vi "JKISM++ State Table - DebugTool.vi"() -> ()   [LabVIEW 2014]
uses:
  _Support/Typedef/_JKISM Current State.ctl
  _Polymophic/Add State(s) to Queue By BOOL(Element).vi
  _Support/GlobalEvent/FGV-GlobalEventRef.vi
  <resource>/dialog/lvconfig.llb/LV Config Write Numeric (I32).vi
  <resource>/dialog/lvconfig.llb/LV Config Read Numeric (I32).vi
  _Support/jkism-tool-support.lvlib
  JKI State Machine++.lvlib
panel:
  in  "Clear JKISM":bool
  out "Dashboard":T1(array[cluster])
  out "Table Control":string[][](table)
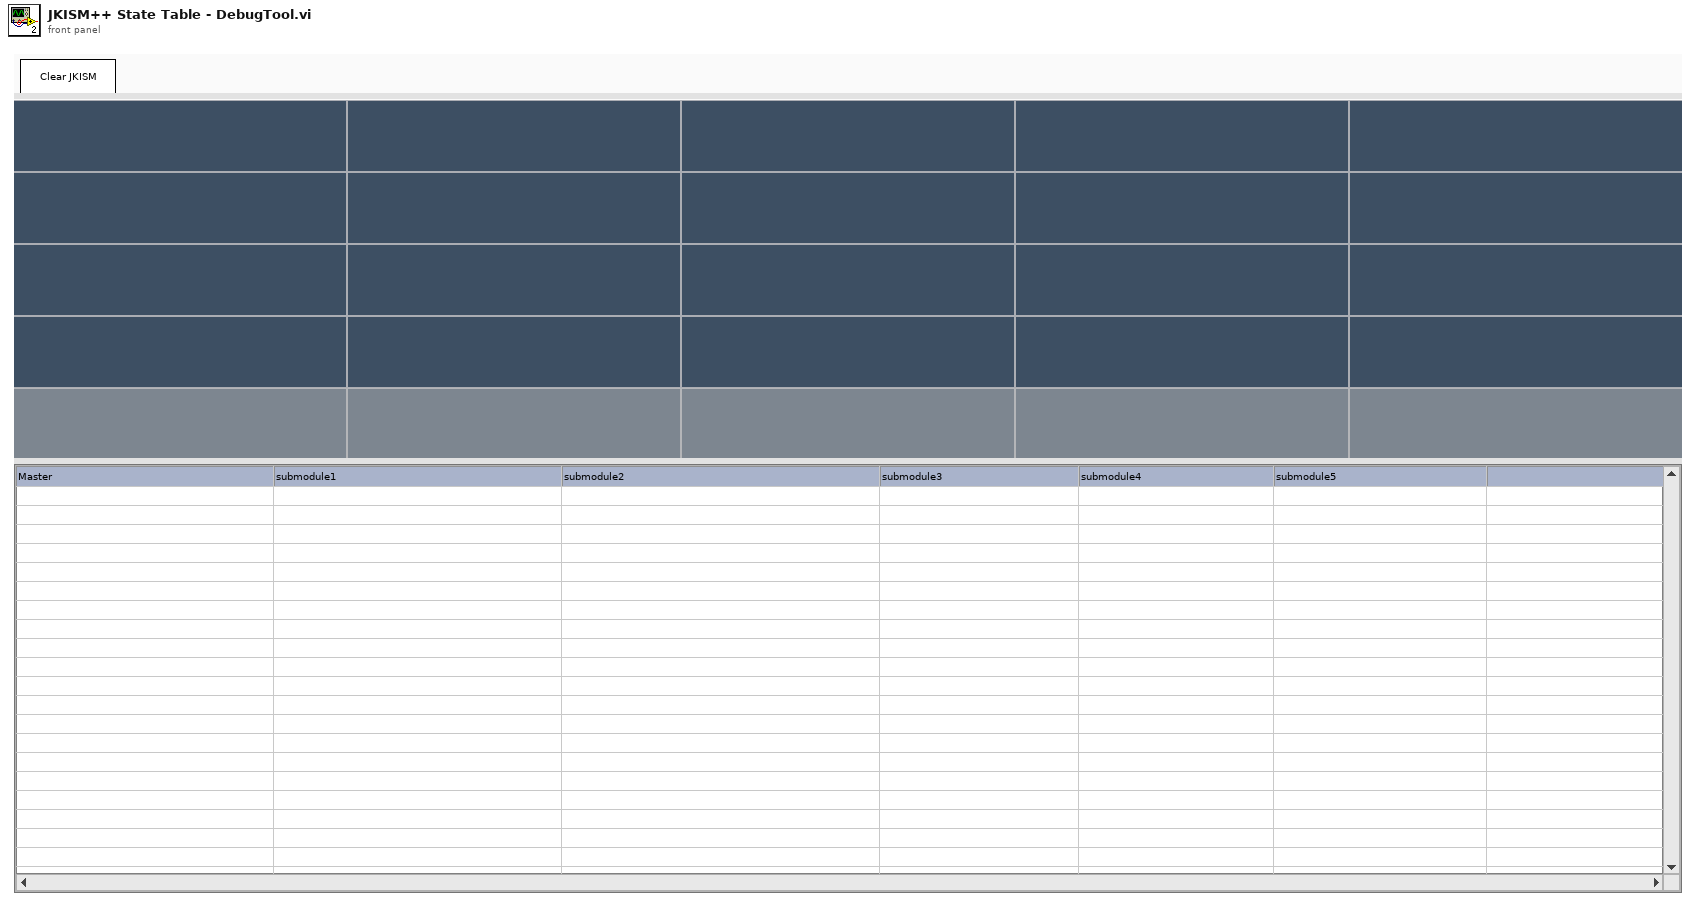
[diagram p1: front panel]
types:
  T1 = cluster{"Label":string, "Value":string, "String":string}[][]
  T2 = enum32{"Invalid", "Standard", "Closed", "Hidden", "Minimized", "Maximized"}
  T3 = enum32{"invalid app kind", "Development System", "Run Time System", "Student Edition", "Embedded LabVIEW", "Evaluation", "Custom"}
  T4 = typedef "JKI State Machine++.lvlib/_JKISM Current State.ctl" = cluster{"Name(\"\" to use uuid)":string, "Current State":string, "Arguments":string, "Argument - State":string, "From Who":string, "Complete(T)/Start(F)":bool}
  T5 = cluster{"Label":string, "Value":string, "String":string}
  T6 = cluster{"Core":cluster{"Current VI Reference":refnum<vi>, "Close Panel on Exit?":bool}, "Global-DataTable":string[][], "NumCols":i16, "NumRows":i16, "JKISM Global Log Event":refnum<user-event>, "Log":T4, "JKISM Names":string[]}
  T7 = cluster{"Current VI Reference":refnum<vi>, "Close Panel on Exit?":bool}
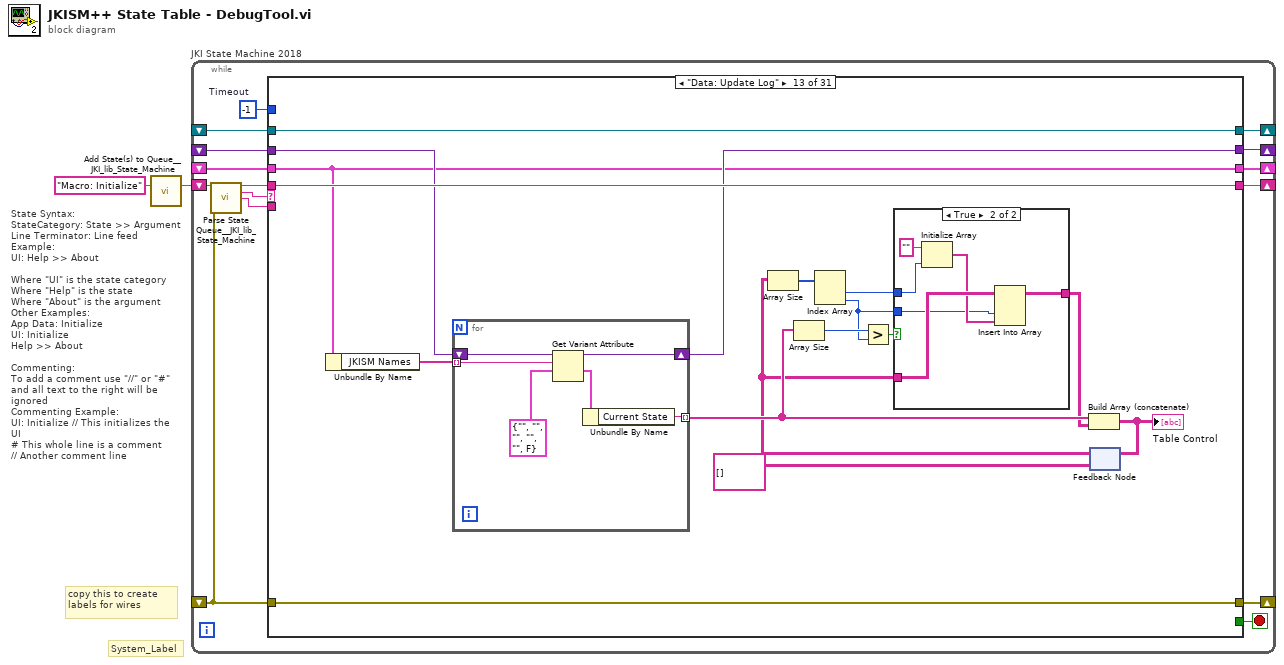
[diagram p0: block diagram]
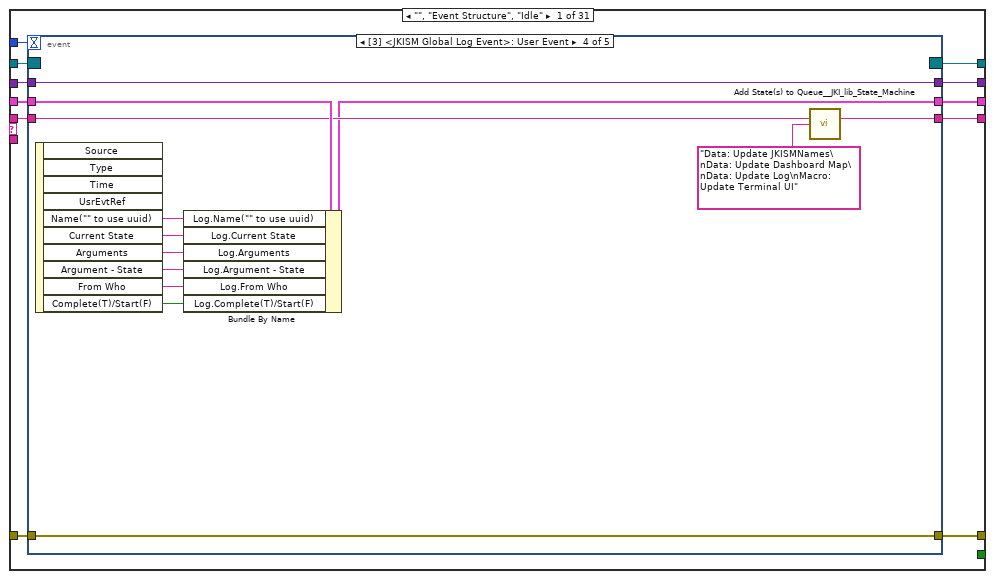
[diagram p2: hidden frame]
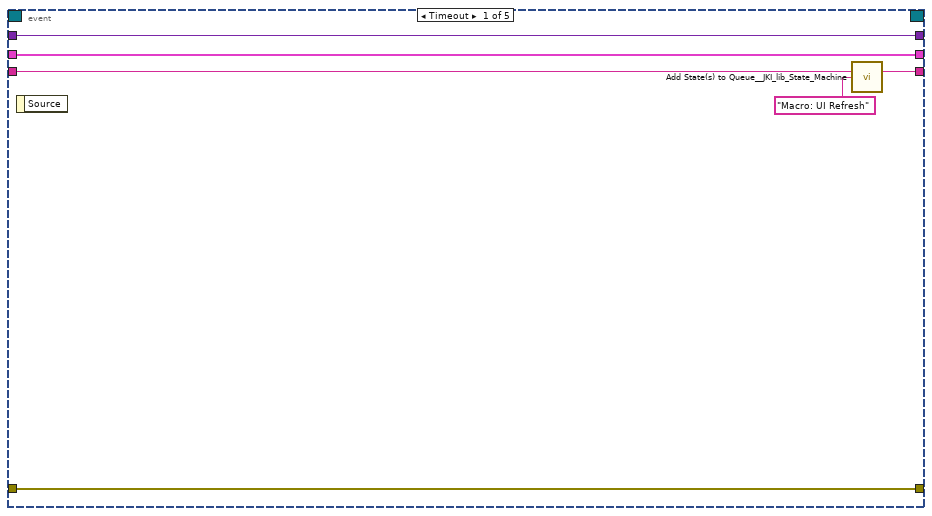
[diagram p3: hidden frame]
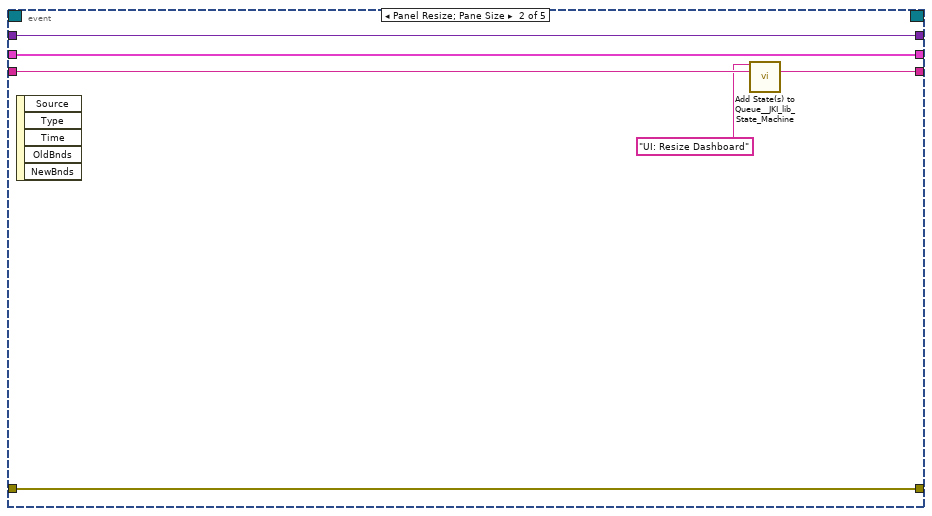
[diagram p4: hidden frame]
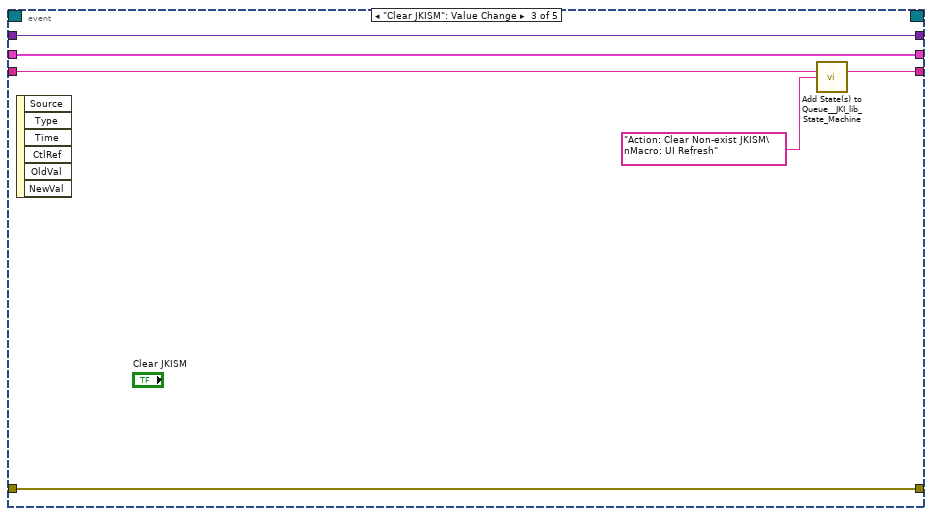
[diagram p5: hidden frame]
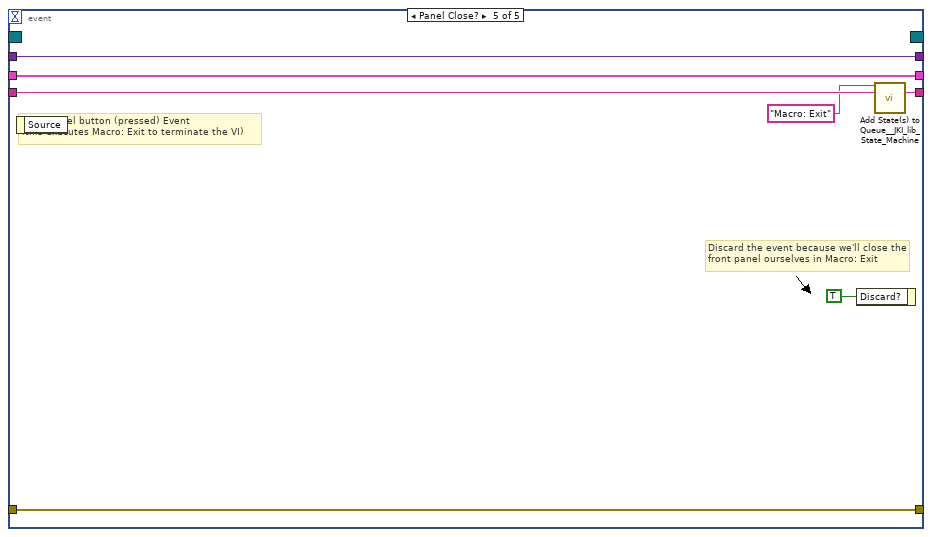
[diagram p6: hidden frame]
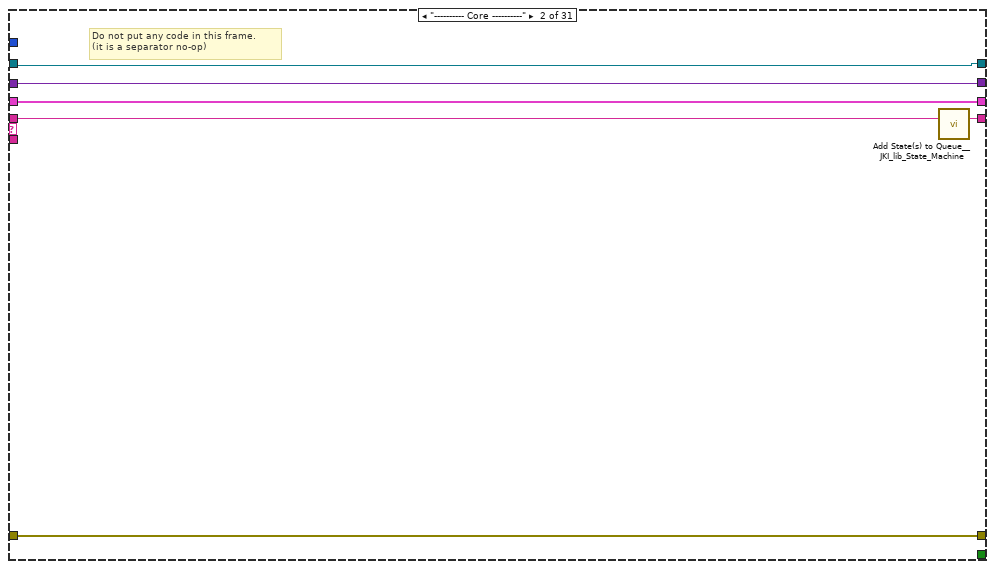
[diagram p7: hidden frame]
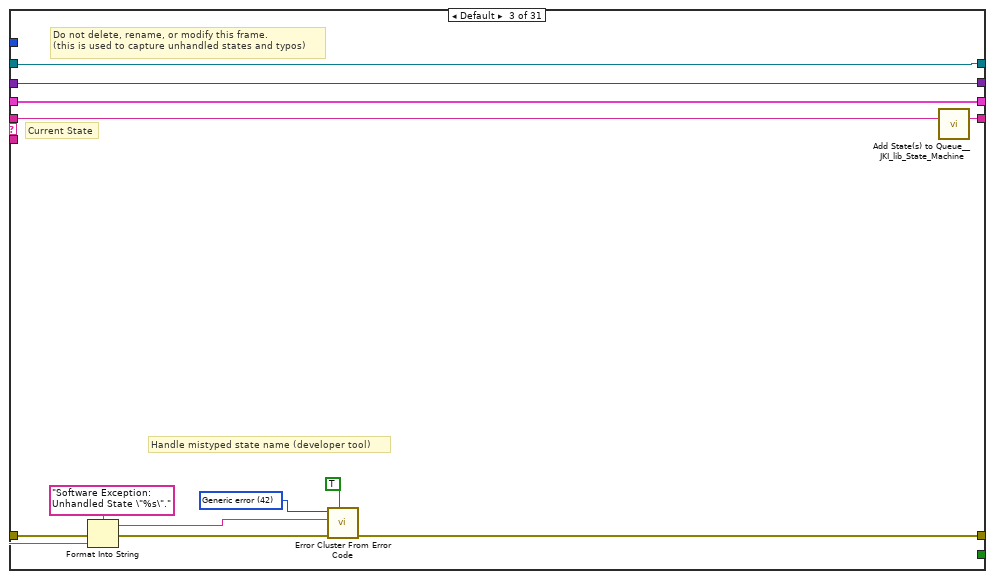
[diagram p8: hidden frame]
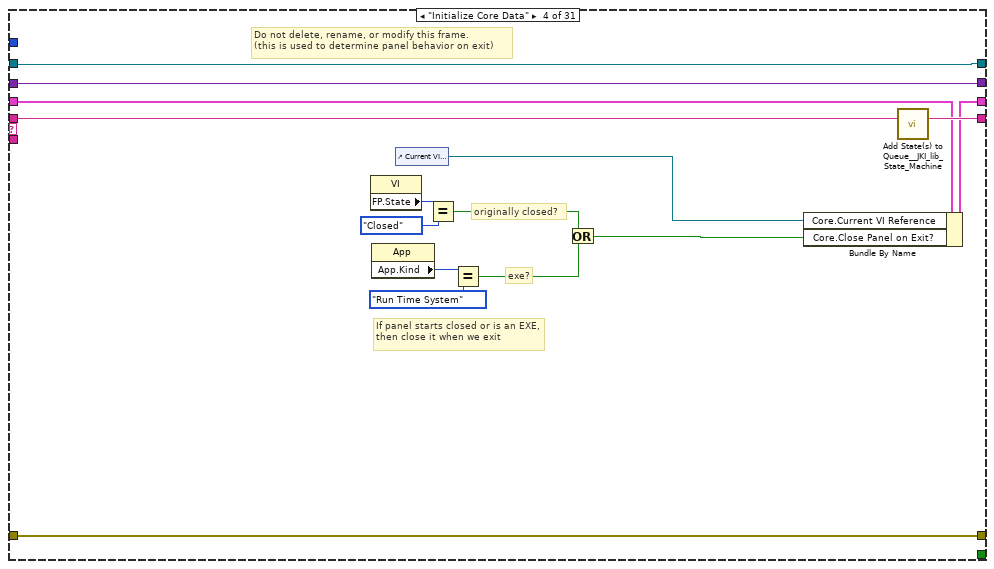
[diagram p9: hidden frame]
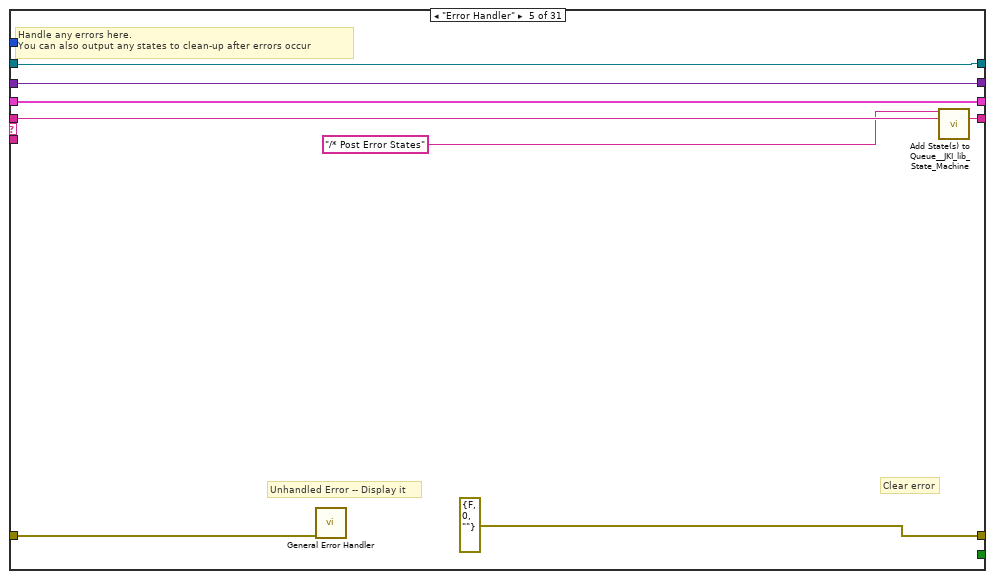
[diagram p10: hidden frame]
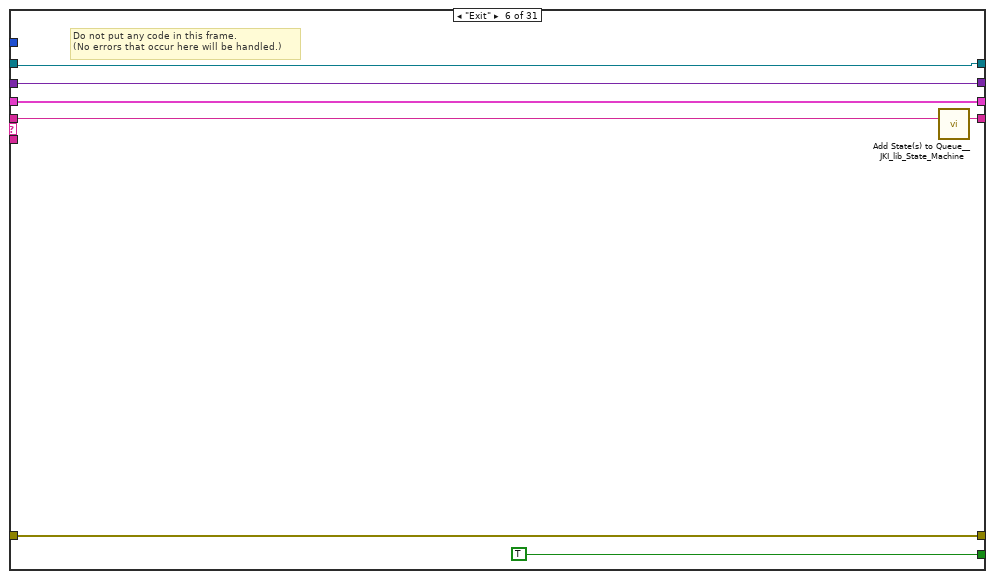
[diagram p11: hidden frame]
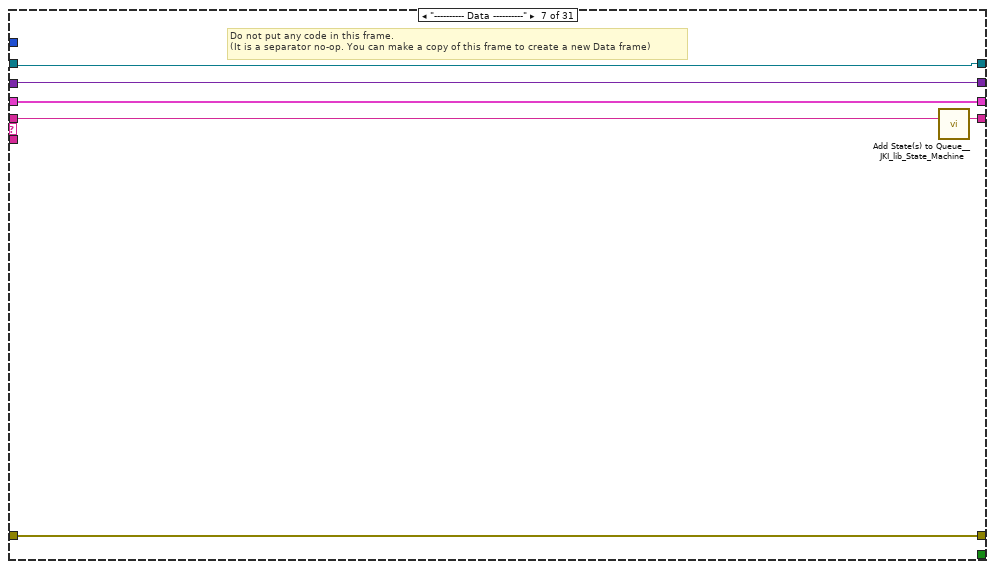
[diagram p12: hidden frame]
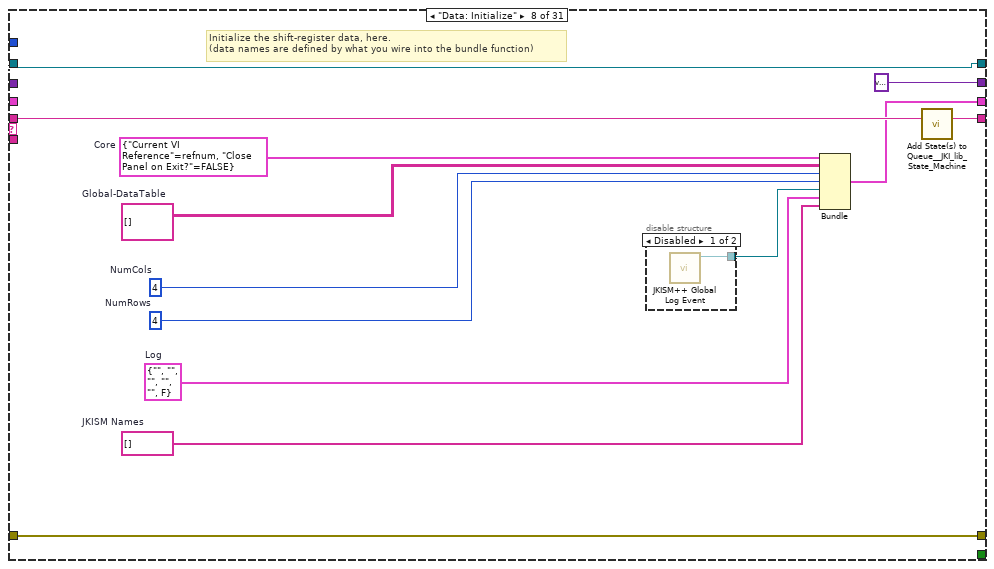
[diagram p13: hidden frame]
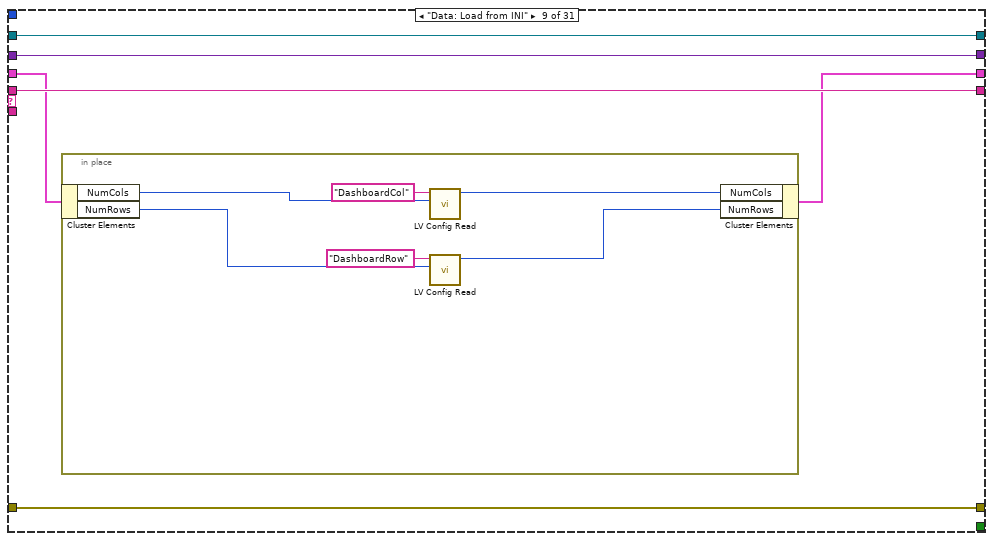
[diagram p15: hidden frame]
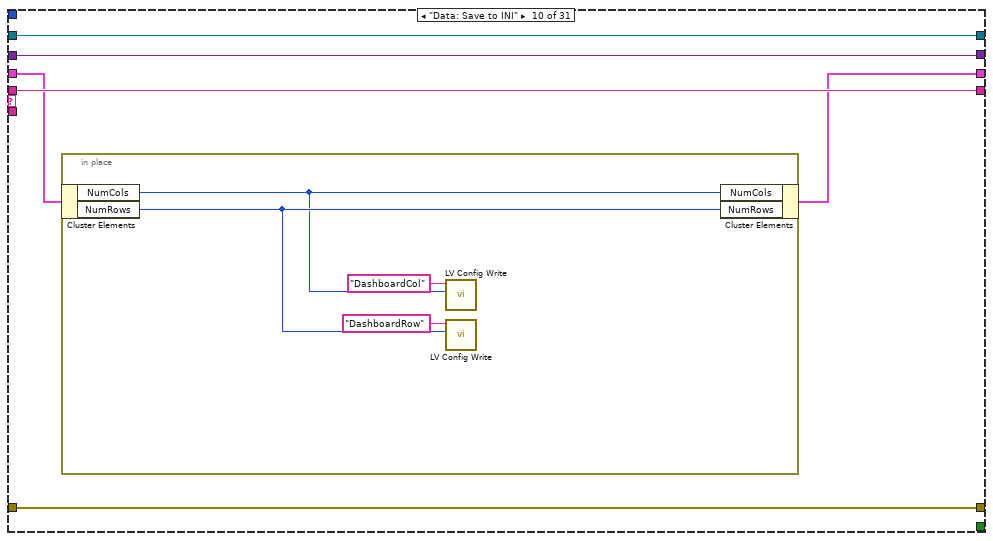
[diagram p16: hidden frame]
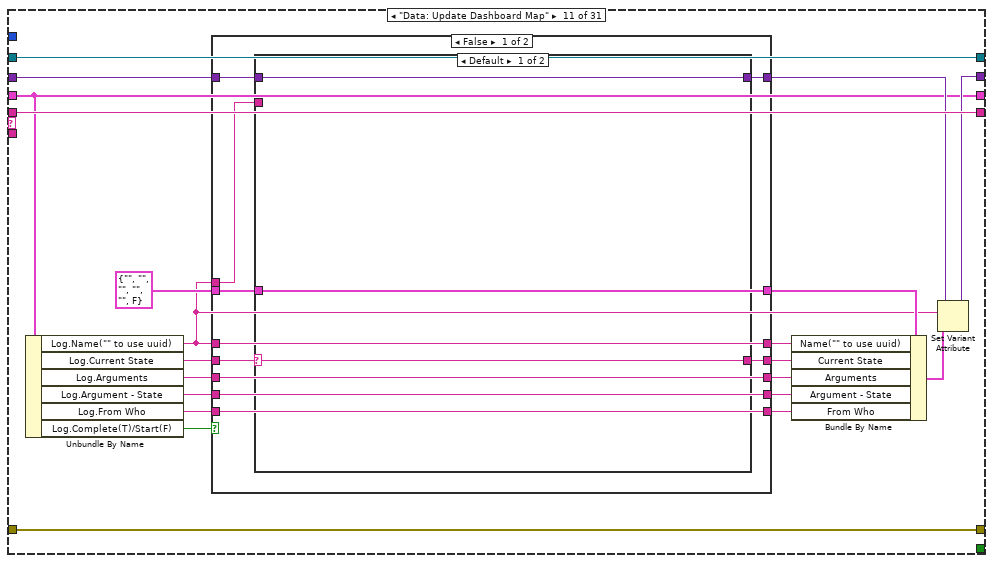
[diagram p17: hidden frame]
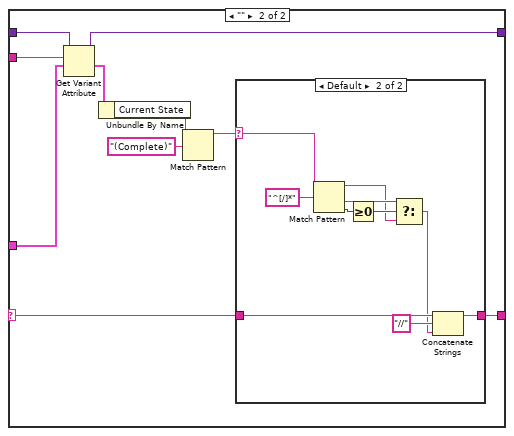
[diagram p18: hidden frame]
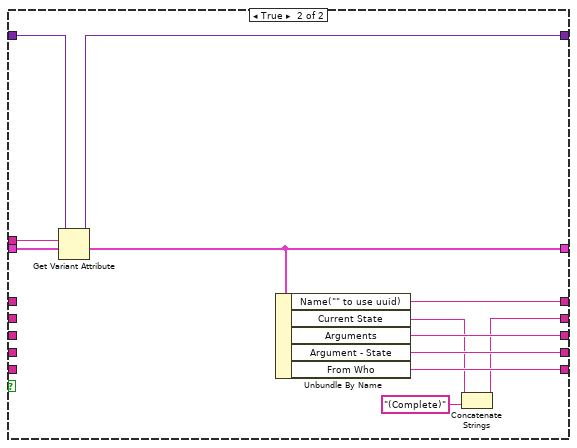
[diagram p20: hidden frame]
diagram:
  # "State Syntax:\nStateCategory: State >> Argument\nLine Terminator: Line feed\nExample:\nUI: Help >> About\n\nWhere \"UI\" is the state category\nWhere \"Help\" is the state\nWhere \"About\" is the argument\nOther Examples:\nApp Data: Initialize\nUI: Initialize\nHelp >> About\n\nCommenting:\nTo add a comment use \"//\" or \"#\" and all text to the right will be ignored\nCommenting Example:\nUI: Initialize // This initializes the UI\n# This whole line is a comment\n// Another comment line"
  # "copy this to create labels for wires"
  # "System_Label"
  n1 = call <vilib>:"Add State(s) to Queue__JKI_lib_State_Machine.vi"("State(s) in (\"\")"="Macro: Initialize") -> ("States Out"=w1:string)  [unwired: 14 in]
  n2 = while "JKI State Machine 2018" {
    shift-right: [w10] -> _
    shift-left: _ -> [w9]
    shift-right: [w13] -> _
    shift-left: _ -> [w7]
    shift-right: [w12] -> _
    shift-left: w1 -> [w14]
    shift-right: [w6] -> _
    shift-left: _ -> [w5]
    shift-right: [w4] -> _
    shift-left: _ -> [w3]
    stop <- w11 stop-if-true
    w8 = -1  # Timeout
    n3 = call <vilib>:"Parse State Queue__JKI_lib_State_Machine.vi"("State Queue"=w14, "Error In (no error)"=w7) -> ("Remaining States"=w16:string, "Current State"=w17:string, "Arguments"=w15:string)  [unwired: 11 in]
    n4 = case shown="\"Data: Update Log\"" w17 {
      selector: w17 -> [_ _ w75 _ _ _ _ _ _ _ _ _ _ _ _ _ _ _ _ _ _ _ _ _ _ _ _ _ _ _ _]
      tunnel: w16 -> [w28 w72 w79 w100 w108 w115 w121 w134 w140 w152 w177 w234 w257 w280 w286 w295 w307 w320 w397 w412 w423 w428 w436 w444 w451 w458 w466 w473 w486 w490 w501]
      tunnel: w15 -> [_ _ _ _ _ _ _ _ _ _ _ _ _ _ _ _ w302 w314 _ _ _ _ _ _ _ _ _ _ _ _ _]
      tunnel: w9 -> [w26 w69 w77 w93 w105 w113 w118 _ w139 w151 w164 w228 w253 w275 w283 w291 w305 w316 w393 w409 w420 w427 w435 w440 w448 w455 w461 w470 w483 w489 w500]
      tunnel: [w25 w70 w81 w97 errorcluster {"status"=FALSE, "code"=0, "source"=""} ("error out") w112 w119 w130 w141 w153 w178 w235 w258 w274 w284 w293 w303 w317 w394 w410 w424 w429 w437 w445 w449 w456 w464 w471 w484 w491 w502] -> w13
      tunnel: w7 -> [w24 w70 w80 w97 w104 w112 w119 w130 w141 w153 w178 w235 w258 w277 w284 w293 w304 w318 _ w410 w424 w429 w437 w445 w449 w456 w464 w471 w484 w491 w502]
      tunnel: [w27 w71 w78 w99 w107 w114 w120 w133 w140 w152 w177 w226 w257 w279 w285 w294 w306 w319 w396 w411 w423 w428 w436 w444 w450 w457 w465 w472 w485 w490 w501] -> w12
      tunnel: [_ _ _ _ _ TRUE _ _ _ _ _ _ _ _ _ _ _ _ _ _ _ _ _ _ _ _ _ _ _ _ _] -> w11
      tunnel: [w23 w69 w77 w98 w105 w113 w118 w132 w138 w150 w164 w227 w253 w275 w283 w291 w305 w316 w393 w409 w420 w427 w431 w440 w448 w455 w461 w470 w483 w489 w500] -> w10
      tunnel: w8 -> [w22 _ _ _ _ _ _ _ _ _ _ _ _ _ _ _ _ _ _ _ _ _ _ _ _ _ _ _ _ _ _]
      tunnel: [w20 w68 w74 w87 w102 w110 w117 variant w137 w149 w165 w232 w254 w273 w282 w288 w301 w313 w390 w404 w422 w426 w434 w443 w447 w453 w460 w468 w476 w488 w496] -> w6
      tunnel: w5 -> [w21 w68 w74 w87 w102 w110 w117 _ w137 w149 w166 w230 w255 w273 w282 w288 w301 w313 w390 w403 w422 w426 w434 w443 w447 w453 w460 w468 w476 w488 w498]
      tunnel: [w18 w67 w73 w86 w101 w109 w116 w125 w136 w148 w176 w233 w256 w272 w281 w287 w300 w312 w389 w400 w421 w425 w432 w442 w446 w452 w459 w467 w475 w487 w499] -> w4
      tunnel: w3 -> [w19 w67 w73 w86 w101 w109 w116 w125 w136 w148 w176 w233 w256 w272 w281 w287 w300 w312 w389 w400 w421 w425 _ w442 w446 w452 w459 w467 w475 w487 w499]
      frame "", "Event Structure", "Idle" {
        n5 = event shown="[3] <JKISM Global Log Event>: User Event" {
          selector: w19 -> [_ _ _ _ _]
          dyn-events: [_ _ _ _ _] -> w18
          timeout: w22 -> [_ _ _ _ _]
          tunnel: w28 -> [w34 w37 w43 w54 w66]
          tunnel: [w33 w38 w42 w58 w65] -> w27
          tunnel: w26 -> [w31 w39 w45 w55 w64]
          tunnel: [w32 w40 w46 w59 w61] -> w25
          tunnel: w24 -> [w32 w40 w46 w59 w61]
          tunnel: [w31 w39 w45 w53 w64] -> w23
          tunnel: w21 -> [w29 w35 w44 w56 w60]
          tunnel: [w29 w35 w44 w56 w60] -> w20
          event Timeout {
            n6 = event-data() -> ()  [unwired: 1 in, 1 out]
            n7 = call <vilib>:"Add State(s) to Queue__JKI_lib_State_Machine.vi"("State(s) in (\"\")"=w34, "State(s) at Back (\"\")"="Macro: UI Refresh" ("State(s) in Front (\"\")")) -> ("States Out"=w33:string)  [unwired: 13 in]
          }
          event Panel Resize; Pane Size {
            n8 = event-data() -> ()  [unwired: 1 in, 5 out]
            n9 = call <vilib>:"Add State(s) to Queue__JKI_lib_State_Machine.vi"("State(s) in Front (\"\")"="UI: Resize Dashboard" ("State(s) in Front (\"\")"), "State(s) in (\"\")"=w37) -> ("States Out"=w38:string)  [unwired: 13 in]
          }
          event "Clear JKISM": Value Change {
            n10 = event-data() -> ()  [unwired: 1 in, 6 out]
            n11 = call <vilib>:"Add State(s) to Queue__JKI_lib_State_Machine.vi"("State(s) in (\"\")"=w43, "State(s) at Back (\"\")"="Action: Clear Non-exist JKISM\nMacro: UI Refresh" ("State(s) at Back (\"\")")) -> ("States Out"=w42:string)  [unwired: 13 in]
          }
          event User Event {
            n12 = event-data() -> ("Name(\"\" to use uuid)"=w47:string, "Current State"=w48:string, "Arguments"=w49:string, "Argument - State"=w50:string, "From Who"=w51:string, "Complete(T)/Start(F)"=w52:bool)  [unwired: 1 in, 4 out]
            n13 = Bundle By Name(cluster=w55, "Log.Name(\"\" to use uuid)"=w47, "Log.Current State"=w48, "Log.Arguments"=w49, "Log.Argument - State"=w50, "Log.From Who"=w51, "Log.Complete(T)/Start(F)"=w52) -> (w53:T6)
            n14 = call <vilib>:"Add State(s) to Queue__JKI_lib_State_Machine.vi"("State(s) in (\"\")"=w54, "State(s) at Back (\"\")"="Data: Update JKISMNames\nData: Update Dashboard Map\nData: Update Log\nMacro: Update Terminal UI" ("State(s) at Back (\"\")")) -> ("States Out"=w58:string)  [unwired: 13 in]
          }
          event Panel Close? {
            # "Discard the event because we'll close the front panel ourselves in Macro: Exit"
            # "Close Panel button (pressed) Event\n(this executes Macro: Exit to terminate the VI)"
            n15 = event-data() -> ()  [unwired: 1 in, 1 out]
            n16 = event-data("Discard?"=TRUE) -> ()  [unwired: 1 in, 1 out]
            n17 = call <vilib>:"Add State(s) to Queue__JKI_lib_State_Machine.vi"("State(s) in Front (\"\")"="Macro: Exit", "State(s) in (\"\")"=w66) -> ("States Out"=w65:string)  [unwired: 13 in]
          }
        }
      }
      frame "---------- Core ----------" {
        # "Do not put any code in this frame.\n(it is a separator no-op)"
        n18 = call <vilib>:"Add State(s) to Queue__JKI_lib_State_Machine.vi"("State(s) in (\"\")"=w72) -> ("States Out"=w71:string)  [unwired: 14 in]
      }
      frame Default {
        w84 = 42 items=["No error", "Argument error", "Memory is full", "Out of zone", "End of file", "File already open", "Generic file I/O error", "File not found", "File permission error", "Disk is full", "Duplicate path", "Too many files open", "System feature not enabled", "Resource file not found", "Cannot add resource", "Resource not found", "Image not found", "Image memory error", "Pen does not exist", "Config type invalid", "Config token not found", "Config parse error", "Config memory error", "Bad external code format", "Bad external code offset", "External code not present", "Null window", "Destroy window error", "Null menu", "Print aborted", "Bad print record", "Print driver error", "Windows error during printing", "Memory error during printing", "Print dialog error", "Generic print error", "Invalid device refnum", "Device not found", "Device parameter error", "Device unit error", "Cannot open device", "Device call aborted", "Generic error", "Cancelled by user", "Object ID too low", "Object ID too high", "Object not in heap", "Unknown heap", "Unknown object (invalid DefProc)", "Unknown object (DefProc not in table)", "Message out of range", "Invalid (null) method", "Unknown message", "Manager call not supported", "Bad address", "Network operation in progress", "Network operation timed out", "Connection is busy", "Network attribute not supported", "Network error", "Address in use", "System out of memory", "Connection aborted", "Connection refused", "Not connected", "Already connected", "Connection closed", "Initialization error (interapplication manager)", "Bad occurrence", "Wait on unbound occurrence handler", "Occurrence queue overflow", "Datalog type conflict", "Unused", "Unrecognized type (interapplication manager)", "Memory corrupt", "Failed to make temporary DLL", "Old CIN version", "Drag socket not found", "Failed to load drop-object", "Failed to register OLE object", "Failed to release OLE object", "Format specifier type mismatch", "Unknown format specifier", "Too few format specifiers", "Too many format specifiers", "Scan failed", "Newer CIN version", "Error converting to variant", "Runtime menu error", "Password tampered", "Variant attribute not found", "Incompatible variant data type", "Event data is not available", "Event Store is not present", "Occurrence is not found", "Event Queue is not created", "Event info is not available", "Refnum passed is NULL", "Error retrieving Class GUID", "Error retrieving CoClass GUID", "Error retrieving TypeLib GUID.", "Bad built application magic bytes.", "Specific driver is different from the specific driver associated with the Logical Name.", "There is no session opened to the class driver.", "Max Error", "MAX - Error with config objects", "MAX - Error loading configuration", "MAX - Group not supported"]
        # "Current State"
        # "Do not delete, rename, or modify this frame.\n(this is used to capture unhandled states and typos)"
        # "Handle mistyped state name (developer tool)"
        n19 = Format Into String(format string="Software Exception: Unhandled State \"%s\"." ("message"), error in=w80, w75) -> (resulting string=w83:string, error out=w82:errorcluster)  [unwired: 1 in]
        n20 = call <vilib>:"Error Cluster From Error Code.vi"("show call chain? (False)"=TRUE, "error in (no error)"=w82, "error message (\"\")"=w83, "error code (0)"=w84) -> ("error out"=w81:errorcluster)  [unwired: 5 in]
        n21 = call <vilib>:"Add State(s) to Queue__JKI_lib_State_Machine.vi"("State(s) in (\"\")"=w79) -> ("States Out"=w78:string)  [unwired: 14 in]
      }
      frame "Initialize Core Data" {
        # "Do not delete, rename, or modify this frame.\n(this is used to determine panel behavior on exit)"
        # "originally closed?"
        # "exe?"
        # "If panel starts closed or is an EXE, then close it when we exit"
        n22 = property class="VI"() -> ("FP.State"=w90:T2)  [unwired: 2 in, 2 out]
        n23 = property class="App"() -> ("App.Kind"=w96:T3)  [unwired: 2 in, 2 out]
        n24 = control-ref of="Current VI Reference"() -> (w91:refnum<vi>)
        n25 = Equal?(x=w90, y=T2."Closed" ("Front Panel Window:State")) -> (x = y?=w88:bool)
        n26 = Equal?(x=w96, y=T3."Run Time System" ("Application:Kind")) -> (x = y?=w94:bool)
        n27 = Or(x=w88, y=w94) -> (x .or. y?=w92:bool)
        n28 = Bundle By Name(cluster=w93, "Core.Current VI Reference"=w91, "Core.Close Panel on Exit?"=w92) -> (w98:T6)
        n29 = call <vilib>:"Add State(s) to Queue__JKI_lib_State_Machine.vi"("State(s) in (\"\")"=w100) -> ("States Out"=w99:string)  [unwired: 14 in]
      }
      frame "Error Handler" {
        # "Unhandled Error -- Display it"
        # "Handle any errors here.\nYou can also output any states to clean-up after errors occur"
        # "Clear error"
        n30 = call <vilib>:"General Error Handler.vi"("error in (no error)"=w104) -> ()  [unwired: 10 in, 5 out]
        n31 = call <vilib>:"Add State(s) to Queue__JKI_lib_State_Machine.vi"("State(s) in Front (\"\")"="/* Post Error States", "State(s) in (\"\")"=w108) -> ("States Out"=w107:string)  [unwired: 13 in]
      }
      frame "Exit" {
        # "Do not put any code in this frame.\n(No errors that occur here will be handled.)"
        n32 = call <vilib>:"Add State(s) to Queue__JKI_lib_State_Machine.vi"("State(s) in (\"\")"=w115) -> ("States Out"=w114:string)  [unwired: 14 in]
      }
      frame "---------- Data ----------" {
        # "Do not put any code in this frame.\n(It is a separator no-op. You can make a copy of this frame to create a new Data frame)"
        n33 = call <vilib>:"Add State(s) to Queue__JKI_lib_State_Machine.vi"("State(s) in (\"\")"=w121) -> ("States Out"=w120:string)  [unwired: 14 in]
      }
      frame "Data: Initialize" {
        w122 = string[] []  # JKISM Names
        w123 = T4 {"Name(\"\" to use uuid)"="", "Current State"="", "Arguments"="", "Argument - State"="", "From Who"="", "Complete(T)/Start(F)"=FALSE}  # Log
        w128 = i16 4  # NumCols
        w127 = i16 4  # NumRows
        w129 = string[][] []  # Global-DataTable
        w131 = T7 {"Current VI Reference"=refnum, "Close Panel on Exit?"=FALSE}  # Core
        # "Initialize the shift-register data, here.\n(data names are defined by what you wire into the bundle function)"
        n34 = disable-structure shown="Disabled" {
          disable-tunnel: [w135 _] -> w124
          frame Disabled {
            n35 = call "JKISM++ Global Log Event.vi"() -> ("JKISM Global Log Event"=w135:refnum<user-event>)  [unwired: 10 in, 1 out]
          }
          frame Enabled {
          }
        }
        n36 = Bundle("Core"=w131, "Global-DataTable"=w129, "NumCols"=w128, "NumRows"=w127, "JKISM Global Log Event"=w124, "Log"=w123, "JKISM Names"=w122) -> (w132:T6)  [unwired: 1 in]
        n37 = call <vilib>:"Add State(s) to Queue__JKI_lib_State_Machine.vi"("State(s) in (\"\")"=w134) -> ("States Out"=w133:string)  [unwired: 14 in]
      }
      frame "Data: Load from INI" {
        n38 = in-place {
          n39 = in-place-cluster #1(w139) -> ("NumCols"=w143:i16, "NumRows"=w146:i16)
          n40 = call-poly <resource>:"LV Config Read.vi"("default value"=w143, "key"="DashboardCol") -> ("value"=w142:i32)  [unwired: 3 in, 2 out]
          n41 = call-poly <resource>:"LV Config Read.vi"("default value"=w146, "key"="DashboardRow") -> ("value"=w145:i32)  [unwired: 3 in, 2 out]
          n42 = in-place-cluster #1("NumCols"=w142, "NumRows"=w145) -> (w138:T6)
        }
      }
      frame "Data: Save to INI" {
        n43 = in-place {
          n44 = in-place-cluster #2(w151) -> ("NumCols"=w154:i16, "NumRows"=w155:i16)
          n45 = call-poly <resource>:"LV Config Write.vi"("value"=w154, "key"="DashboardCol") -> ()  [unwired: 5 in, 1 out]
          n46 = call-poly <resource>:"LV Config Write.vi"("value"=w155, "key"="DashboardRow") -> ()  [unwired: 5 in, 1 out]
          n47 = in-place-cluster #2("NumCols"=w154, "NumRows"=w155) -> (w150:T6)
        }
      }
      frame "Data: Update Dashboard Map" {
        n48 = Unbundle By Name(w164) -> ("Log.Name(\"\" to use uuid)"=w158:string, "Log.Current State"=w163:string, "Log.Arguments"=w162:string, "Log.Argument - State"=w161:string, "Log.From Who"=w160:string, "Log.Complete(T)/Start(F)"=w159:bool)
        n49 = case shown="False" w159 {
          tunnel: w166 -> [w184 w223]
          tunnel: [w183 w222] -> w174
          tunnel: T4 {"Name(\"\" to use uuid)"="", "Current State"="", "Arguments"="", "Argument - State"="", "From Who"="", "Complete(T)/Start(F)"=FALSE} ("Cross JKI State Machine Data") -> [w181 w221]
          tunnel: w158 -> [w182 w220]
          tunnel: w160 -> [w188 _]
          tunnel: [w188 w219] -> w172
          tunnel: w161 -> [w187 _]
          tunnel: [w187 w218] -> w171
          tunnel: w162 -> [w186 _]
          tunnel: [w186 w217] -> w170
          tunnel: w163 -> [w180 _]
          tunnel: [w179 w212] -> w169
          tunnel: w158 -> [w185 _]
          tunnel: [w185 w214] -> w168
          tunnel: [w181 w215] -> w167
          frame False {
            n50 = case shown="Default" w180 {
              selector: w180 -> [w189 w192]
              tunnel: w184 -> [w190 w200]
              tunnel: [w190 w199] -> w183
              tunnel: w182 -> [_ w198]
              tunnel: w181 -> [_ w196]
              tunnel: [w189 w191] -> w179
              frame Default {
              }
              frame "" {
                n51 = Get Variant Attribute(Variant=w200, name=w198, default value (empty Variant)=w196) -> (duplicate Variant=w199:variant, value=w197:T4)  [unwired: 1 in, 2 out]
                n52 = Unbundle By Name(w197) -> ("Current State"=w195:string)
                n53 = Match Pattern(string=w195, regular expression="(Complete)") -> (before substring=w193:string)  [unwired: 1 in, 3 out]
                n54 = case shown="Default" w193 {
                  selector: w193 -> [_ w207]
                  tunnel: w192 -> [w201 w211]
                  tunnel: [w201 w210] -> w191
                  frame "" {
                  }
                  frame Default {
                    n55 = Match Pattern(string=w207, regular expression="^[/]*") -> (before substring=w202:string, after substring=w204:string, offset past match=w206:i32)  [unwired: 1 in, 1 out]
                    n56 = Greater Or Equal To 0?(x=w206) -> (x >= 0?=w205:bool)
                    n57 = Select(t=w204, s=w205, f=w202) -> (s? t:f=w203:string)
                    n58 = Concatenate Strings(w211, "//" ("string"), w203) -> (w210:string)
                  }
                }
              }
            }
          }
          frame True {
            n59 = Get Variant Attribute(Variant=w223, name=w220, default value (empty Variant)=w221) -> (duplicate Variant=w222:variant, value=w215:T4)  [unwired: 1 in, 2 out]
            n60 = Unbundle By Name(w215) -> ("Name(\"\" to use uuid)"=w214:string, "Current State"=w213:string, "Arguments"=w217:string, "Argument - State"=w218:string, "From Who"=w219:string)
            n61 = Concatenate Strings(w213, "(Complete)" ("string")) -> (w212:string)
          }
        }
        n62 = Bundle By Name(cluster=w167, "Name(\"\" to use uuid)"=w168, "Current State"=w169, "Arguments"=w170, "Argument - State"=w171, "From Who"=w172) -> (w175:T4)
        n63 = Set Variant Attribute(Variant=w174, name=w158, value=w175) -> (Variant out=w165:variant)  [unwired: 1 in, 2 out]
      }
      frame "Data: Update JKISMNames" {
        n64 = Unbundle By Name(w228) -> ("Log.Name(\"\" to use uuid)"=w229:string)
        n65 = Get Variant Attribute(Variant=w230, name=w229, default value (empty Variant)=T4 {"Name(\"\" to use uuid)"="", "Current State"="", "Arguments"="", "Argument - State"="", "From Who"="", "Complete(T)/Start(F)"=FALSE} ("Cross JKI State Machine Data")) -> (duplicate Variant=w232:variant, found=w225:bool)  [unwired: 1 in, 2 out]
        n66 = case shown="False" w225 {
          tunnel: w228 -> [w238 w241]
          tunnel: w229 -> [w239 _]
          tunnel: [w236 w241] -> w227
          frame False {
            n67 = Unbundle By Name(w238) -> ("JKISM Names"=w240:string[])
            n68 = Build Array (concatenate)(w240, w239) -> (w237:string[])
            n69 = Bundle By Name(cluster=w238, "JKISM Names"=w237) -> (w236:T6)
          }
          frame True {
          }
        }
        n70 = call-poly "Add State(s) to Queue By BOOL++.vi"("False(\"\")"="UI: Update Column Names" ("TRUE(\"\")"), "Bool"=w225, "State Queue(\"\")"=w234) -> ("State Queue Out"=w226:string)  [unwired: 8 in]
      }
      frame "Data: Update Log" {
        n71 = Unbundle By Name(w253) -> ("JKISM Names"=w252:string[])
        n72 = for {
          shift-right: [w269] -> w254
          shift-left: w255 -> [w270]
          tunnel: w252 -> [w268] mode=indexing
          tunnel: [w266] -> w248 mode=indexing
          n73 = Get Variant Attribute(Variant=w270, name=w268, default value (empty Variant)=T4 {"Name(\"\" to use uuid)"="", "Current State"="", "Arguments"="", "Argument - State"="", "From Who"="", "Complete(T)/Start(F)"=FALSE} ("Cross JKI State Machine Data")) -> (duplicate Variant=w269:variant, value=w267:T4)  [unwired: 1 in, 2 out]
          n74 = Unbundle By Name(w267) -> ("Current State"=w266:string)
        }
        n75 = Array Size(array=w248) -> (size(s)=w247:i32)
        n76 = feedback #3(string[][] []) -> (w246:string[][])
        n77 = Array Size(array=w246) -> (size(s)=w249:i32[])
        n78 = Index Array(array=w249) -> (element #1=w245:i32, element #2=w244:i32)  [unwired: 2 in]
        n79 = Greater?(x=w247, y=w244) -> (0:w242:bool)
        n80 = case shown="True" w242 {
          tunnel: w246 -> [w259 w265]
          tunnel: w245 -> [_ w263]
          tunnel: w244 -> [_ w261]
          tunnel: [w259 w260] -> w243
          frame False {
          }
          frame True {
            n81 = Initialize Array("" ("Current State"), w263) -> (w262:string[])
            n82 = Insert Into Array(array=w265, index (col)=w261, new element=w262) -> (w260:string[][])  [unwired: 1 in]
          }
        }
        n83 = Build Array (concatenate)(w248, w243) -> (w251:string[][])
        "Table Control" <- w251
        n84 = feedback-in #3(w251) -> ()
      }
      frame "Data: Cleanup" {
        # "Cleanup any data and references, here.\n(this is called automatically, by the Macro: Exit)"
        n85 = Unbundle By Name(w275) -> ("Core.Current VI Reference"=w278:refnum<vi>)
        n86 = Close Reference(reference=w278, error in (no error)=w277) -> (error out=w276:errorcluster)
        n87 = Merge Errors(w276) -> (w274:errorcluster)
        n88 = call <vilib>:"Add State(s) to Queue__JKI_lib_State_Machine.vi"("State(s) in (\"\")"=w280) -> ("States Out"=w279:string)  [unwired: 14 in]
      }
      frame "---------- UI ----------" {
        # "Do not put any code in this frame.\n(It is a separator no-op. You can make a copy of this frame to create a new UI frame)"
        n89 = call <vilib>:"Add State(s) to Queue__JKI_lib_State_Machine.vi"("State(s) in (\"\")"=w286) -> ("States Out"=w285:string)  [unwired: 14 in]
      }
      frame "UI: Initialize" {
        # "Initialize the User Interface, here.\n(this is called automatically, by the Macro: Init)"
        n90 = invoke class="VI" method="Default Vals.Reinit All"() -> (error out=w292:errorcluster)  [unwired: 3 in, 2 out]
        n91 = Unbundle By Name(w291) -> ("NumRows"=w290:i16, "NumCols"=w289:i16)
        n92 = flat-sequence {
          tunnel: w292 -> [_]
          tunnel: w290 -> [w297]
          tunnel: w289 -> [w296]
          frame #0 {
            n93 = Initialize Array(T5 {"Label"="", "Value"="", "String"=""} ("Dashboard"), w297, w296) -> (w298:T1)
            n94 = local write "Dashboard"(w298) -> ()
          }
        }
        n95 = call <vilib>:"Add State(s) to Queue__JKI_lib_State_Machine.vi"("State(s) in (\"\")"=w295) -> ("States Out"=w294:string)  [unwired: 14 in]
      }
      frame "UI: Cursor Set" {
        # "Argument"
        # "Set and Unset Cursor Busy.\n(Usage: \"UI: Cursor Set >> Busy|Idle\")"
        n96 = case shown="\"Idle\", Default" w302 {
          tunnel: w304 -> [w309 w311]
          tunnel: [w308 w310] -> w303
          frame "Idle", Default {
            n97 = call <vilib>:"Unset Busy.vi"("error in (no error)"=w309) -> ("error out"=w308:errorcluster)  [unwired: 10 in]
          }
          frame "Busy" {
            n98 = call <vilib>:"Set Busy.vi"("error in (no error)"=w311) -> ("error out"=w310:errorcluster)  [unwired: 9 in, 1 out]
          }
        }
        n99 = call <vilib>:"Add State(s) to Queue__JKI_lib_State_Machine.vi"("State(s) in (\"\")"=w307) -> ("States Out"=w306:string)  [unwired: 14 in]
      }
      frame "UI: Front Panel State" {
        # "Argument"
        # "Set Front Panel Open or Closed\n(Usage: \"UI: Front Panel State >> Open|Close\")"
        n100 = Unbundle By Name(w316) -> ("Core.Current VI Reference"=w315:refnum<vi>)
        n101 = case shown="\"Minimize\", \"Minimized\"" w314 {
          tunnel: w318 -> [w326 w341 w352 w365 w378]
          tunnel: [w328 w342 w354 w367 w380] -> w317
          tunnel: w315 -> [w327 w339 w353 w366 w379]
          frame "Open", "Standard", Default {
            w321 = T2."Standard" ("State")
            n102 = property class="VI"(reference=w327, error in=w326) -> (reference out=w324:refnum<vi>, error out=w325:errorcluster, "FP.State"=w323:T2)
            n103 = Not Equal?(x=w323, y=w321) -> (x != y?=w322:bool)
            n104 = case shown="True" w322 {
              tunnel: [w332 w334] -> w328
              tunnel: w325 -> [w331 w334]
              tunnel: w324 -> [w330 _]
              tunnel: w321 -> [w329 _]
              frame True {
                n105 = invoke class="VI" method="FP.Open"(reference=w330, error in=w331, "Activate"=TRUE, "State"=w329) -> (error out=w332:errorcluster)  [unwired: 1 in, 4 out]
              }
              frame False {
              }
            }
          }
          frame "Close", "Closed" {
            n106 = property class="VI"(reference=w339, error in=w341) -> (reference out=w338:refnum<vi>, error out=w340:errorcluster, "FP.State"=w336:T2)
            n107 = Not Equal?(x=w336, y=T2."Closed" ("Front Panel Window:State")) -> (x != y?=w335:bool)
            n108 = case shown="True" w335 {
              tunnel: [w343 w346] -> w342
              tunnel: w340 -> [w343 w345]
              tunnel: w338 -> [_ w344]
              frame False {
              }
              frame True {
                n109 = invoke class="VI" method="FP.Close"(reference=w344, error in=w345) -> (error out=w346:errorcluster)  [unwired: 1 in, 2 out]
              }
            }
          }
          frame "Hidden", "Hide" {
            w347 = T2."Hidden" ("State")
            n110 = property class="VI"(reference=w353, error in=w352) -> (reference out=w350:refnum<vi>, error out=w351:errorcluster, "FP.State"=w349:T2)
            n111 = Not Equal?(x=w349, y=w347) -> (x != y?=w348:bool)
            n112 = case shown="True" w348 {
              tunnel: [w358 w359] -> w354
              tunnel: w351 -> [w357 w359]
              tunnel: w350 -> [w356 _]
              tunnel: w347 -> [w355 _]
              frame True {
                n113 = invoke class="VI" method="FP.Open"(reference=w356, error in=w357, "State"=w355) -> (error out=w358:errorcluster)  [unwired: 2 in, 4 out]
              }
              frame False {
              }
            }
          }
          frame "Minimize", "Minimized" {
            w360 = T2."Minimized" ("State")
            n114 = property class="VI"(reference=w366, error in=w365) -> (reference out=w363:refnum<vi>, error out=w364:errorcluster, "FP.State"=w362:T2)
            n115 = Not Equal?(x=w362, y=w360) -> (x != y?=w361:bool)
            n116 = case shown="True" w361 {
              tunnel: [w371 w372] -> w367
              tunnel: w364 -> [w370 w372]
              tunnel: w363 -> [w369 _]
              tunnel: w360 -> [w368 _]
              frame True {
                n117 = invoke class="VI" method="FP.Open"(reference=w369, error in=w370, "State"=w368) -> (error out=w371:errorcluster)  [unwired: 2 in, 4 out]
              }
              frame False {
              }
            }
          }
          frame "Maximize", "Maximized" {
            w373 = T2."Maximized" ("State")
            n118 = property class="VI"(reference=w379, error in=w378) -> (reference out=w376:refnum<vi>, error out=w377:errorcluster, "FP.State"=w375:T2)
            n119 = Not Equal?(x=w375, y=w373) -> (x != y?=w374:bool)
            n120 = case shown="True" w374 {
              tunnel: [w384 w385] -> w380
              tunnel: w377 -> [w383 w385]
              tunnel: w376 -> [w382 _]
              tunnel: w373 -> [w381 _]
              frame True {
                n121 = invoke class="VI" method="FP.Open"(reference=w382, error in=w383, "State"=w381) -> (error out=w384:errorcluster)  [unwired: 2 in, 4 out]
              }
              frame False {
              }
            }
          }
        }
        n122 = call <vilib>:"Add State(s) to Queue__JKI_lib_State_Machine.vi"("State(s) in (\"\")"=w320) -> ("States Out"=w319:string)  [unwired: 14 in]
      }
      frame "UI: Resize Dashboard" {
        # "Do not put any code in this frame.\n(It is a separator no-op. You can make a copy of this frame to create a new UI frame)"
        n123 = control-ref of="Dashboard"() -> (w395:refnum<vi>)
        n124 = control-ref of="Pane 3"() -> (w388:refnum<vi>)
        n125 = Unbundle By Name(w393) -> ("NumCols"=w391:i16, "NumRows"=w392:i16)
        n126 = property class="Pane"(reference=w388) -> ("Width"=w387:u32, "Height"=w386:u32)  [unwired: 1 in, 2 out]
        n127 = call "Dashboard Cell2 Array Resize.vi"("Num Columns"=w391, "Num Rows"=w392, "area height"=w386, "area width"=w387, "Array 2"=w395) -> ("error out"=w394:errorcluster)  [unwired: 6 in]
        n128 = call <vilib>:"Add State(s) to Queue__JKI_lib_State_Machine.vi"("State(s) in (\"\")"=w397) -> ("States Out"=w396:string)  [unwired: 14 in]
      }
      frame "UI: Update Dashboard" {
        # "Do not put any code in this frame.\n(It is a separator no-op. You can make a copy of this frame to create a new UI frame)"
        n129 = Get Variant Attribute(Variant=w403) -> (duplicate Variant=w404:variant, names=w402:string[], values=w401:variant[])  [unwired: 3 in, 1 out]
        n130 = Variant To Data(type=T4[] [], Variant=w401) -> (data=w398:T4[])  [unwired: 1 in, 1 out]
        n131 = for {
          tunnel: w402 -> [w417] mode=indexing
          tunnel: [w416] -> w408 mode=indexing
          tunnel: w398 -> [w415] mode=indexing
          n132 = Unbundle By Name(w415) -> ("Current State"=w414:string, "Arguments"=w413:string)  [unwired: 1 out]
          n133 = Bundle By Name(cluster=T5 {"Label"="", "Value"="", "String"=""}, "Label"=w417, "Value"=w414, "String"=w413) -> (w416:T5)
        }
        n134 = Unbundle By Name(w409) -> ("NumRows"=w406:i16, "NumCols"=w405:i16)
        n135 = Reshape Array(w408, w406, w405) -> (→"Dashboard":T1)
        n136 = call <vilib>:"Add State(s) to Queue__JKI_lib_State_Machine.vi"("State(s) in (\"\")"=w412) -> ("States Out"=w411:string)  [unwired: 14 in]
      }
      frame "UI: Update Column Names" {
        n137 = Unbundle By Name(w420) -> ("JKISM Names"=w419:string[])
        n138 = property on="Table Control" class="Tbl (strict)"("Column Headers[]"=w419) -> ()  [unwired: 2 in, 2 out]
      }
      frame "--------- Event ---------" {
      }
      frame "Register User Event" {
        n139 = call "JKISM++ Global Log Event.vi"() -> ("Error out"=w433:errorcluster, "JKISM Global Log Event"=w430:refnum<user-event>)  [unwired: 10 in]
        n140 = register-events(error in=w433, w430) -> (reference out=w432:refnum<event-registration>)  [unwired: 1 in, 1 out]
        n141 = Bundle By Name(cluster=w435, "JKISM Global Log Event"=w430) -> (w431:T6)
      }
      frame "UnRegister User Event" {
        n142 = Unregister For Events(event registration refnum=w442) -> (error out=w441:errorcluster)  [unwired: 1 in]
        n143 = Unbundle By Name(w440) -> ("JKISM Global Log Event"=w439:refnum<user-event>)
        n144 = call "JKISM++ Destroy Global Log Event.vi"("Error in"=w441, "JKISM Global Log Event"=w439) -> ("Error out"=w438:errorcluster)  [unwired: 9 in]
        n145 = call <vilib>:"Clear Errors.vi"("error in (no error)"=w438) -> ()  [unwired: 6 in, 1 out]
      }
      frame "---------- Macro ----------" {
        # "Do not put any code in this frame.\n(It is a separator no-op. You can make a copy of this frame to create a new Macro frame)"
        n146 = call <vilib>:"Add State(s) to Queue__JKI_lib_State_Machine.vi"("State(s) in (\"\")"=w451) -> ("States Out"=w450:string)  [unwired: 14 in]
      }
      frame "Macro: Initialize" {
        # "Initialization Macro\n(This is called once, when the VI starts)"
        n147 = call <vilib>:"Add State(s) to Queue__JKI_lib_State_Machine.vi"("State(s) in Front (\"\")"="Data: Initialize\nInitialize Core Data\nData: Load from INI\nUI: Initialize\nUI: Resize Dashboard\nRegister User Event\n//UI: Front Panel State >> Open", "State(s) in (\"\")"=w458) -> ("States Out"=w457:string)  [unwired: 13 in]
      }
      frame "Macro: UI Refresh" {
        # "Do not put any code in this frame.\n(It is a separator no-op. You can make a copy of this frame to create a new Macro frame)"
        n148 = call <vilib>:"Add State(s) to Queue__JKI_lib_State_Machine.vi"("State(s) at Back (\"\")"="Macro: Update Terminal UI" ("State(s) in Front (\"\")")) -> ("States Out"=w463:string)  [unwired: 14 in]
        n149 = call <vilib>:"Add State(s) to Queue__JKI_lib_State_Machine.vi"("State(s) in Front (\"\")"=w463, "State(s) in (\"\")"=w466) -> ("States Out"=w465:string)  [unwired: 13 in]
      }
      frame "Macro: Update Terminal UI" {
        # "Do not put any code in this frame.\n(It is a separator no-op. You can make a copy of this frame to create a new Macro frame)"
        n150 = call <vilib>:"Add State(s) to Queue__JKI_lib_State_Machine.vi"("State(s) in Front (\"\")"="UI: Update Dashboard" ("State(s) in Front (\"\")"), "State(s) in (\"\")"=w473) -> ("States Out"=w472:string)  [unwired: 13 in]
      }
      frame "Macro: Exit" {
        # "Exit Macro\n(This is called once, when the VI exits)"
        n151 = Unbundle By Name(w483) -> ("Core.Close Panel on Exit?"=w482:bool)
        n152 = Select(t="UI: Front Panel State >> Close", s=w482, f="") -> (s? t:f=w478:string)
        n153 = call <vilib>:"Add State(s) to Queue__JKI_lib_State_Machine.vi"("State(s) in Front (\"\")"="UnRegister User Event" ("State(s) in Front (\"\")"), "State(s) in (\"\")"=w478, "State(s) at Back (\"\")"="Data: Save to INI\nData: Cleanup\nExit") -> ("States Out"=w481:string)  [unwired: 12 in]
        n154 = call <vilib>:"Add State(s) to Queue__JKI_lib_State_Machine.vi"("State(s) in Front (\"\")"=w481, "State(s) in (\"\")"=w486) -> ("States Out"=w485:string)  [unwired: 13 in]
      }
      frame "----- Action ------" {
      }
      frame "Action: Clear Non-exist JKISM" {
        n155 = Get Variant Attribute(Variant=w498) -> (duplicate Variant=w497:variant, names=w495:string[], values=w494:variant[])  [unwired: 3 in, 1 out]
        n156 = Variant To Data(type=T4[] [], Variant=w494) -> (data=w493:T4[])  [unwired: 1 in, 1 out]
        n157 = for {
          shift-right: [w514] -> w496
          shift-left: w497 -> [w515]
          tunnel: w495 -> [w513] mode=indexing
          tunnel: w493 -> [w512] mode=indexing
          n158 = Unbundle By Name(w512) -> ("Current State"=w510:string, "Name(\"\" to use uuid)"=w509:string)
          n159 = Search 1D Array(1D array=string[] ["<Remaining States>", "Exit"], element=w510) -> (index of element=w506:i32)  [unwired: 1 in]
          n160 = Match Pattern(string=w509, regular expression="^-") -> (offset past match=w507:i32)  [unwired: 1 in, 3 out]
          n161 = Greater Or Equal To 0?(x=w506) -> (x >= 0?=w504:bool)
          n162 = Greater Or Equal To 0?(x=w507) -> (x >= 0?=w505:bool)
          n163 = Or(x=w505, y=w504) -> (x .or. y?=w503:bool)
          n164 = case shown="True" w503 {
            tunnel: w515 -> [w516 w519]
            tunnel: [w516 w518] -> w514
            tunnel: w513 -> [_ w517]
            tunnel: w509 -> [_ _]
            tunnel: w510 -> [_ _]
            frame False {
            }
            frame True {
              n165 = Delete Variant Attribute(6:w517, 7:w519) -> (3:w518:variant)  [unwired: 1 in, 2 out]
            }
          }
        }
      }
    }
  }
